vi "init_test_result_table.vi"(10 "Test Table":refnum<vi>, 11 "LED":T1) -> ()   [LabVIEW 2016]
uses:
  <vilib>/Utility/miscctls.llb/LVRowAndColumnTypeDef.ctl
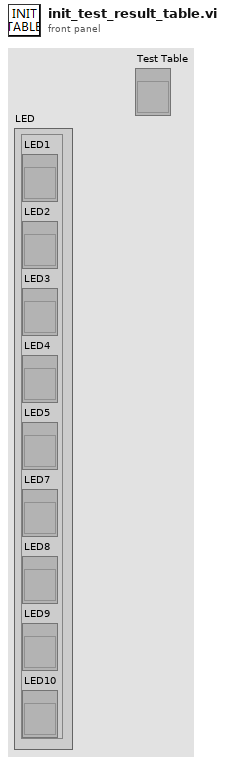
[diagram p1: front panel]
types:
  T1 = cluster{"LED1":refnum<vi>, "LED2":refnum<vi>, "LED3":refnum<vi>, "LED4":refnum<vi>, "LED5":refnum<vi>, "LED7":refnum<vi>, "LED8":refnum<vi>, "LED9":refnum<vi>, "LED10":refnum<vi>}
  T2 = typedef "LVRowAndColumnTypeDef.ctl" = cluster{"Row":i32, "Column":i32}
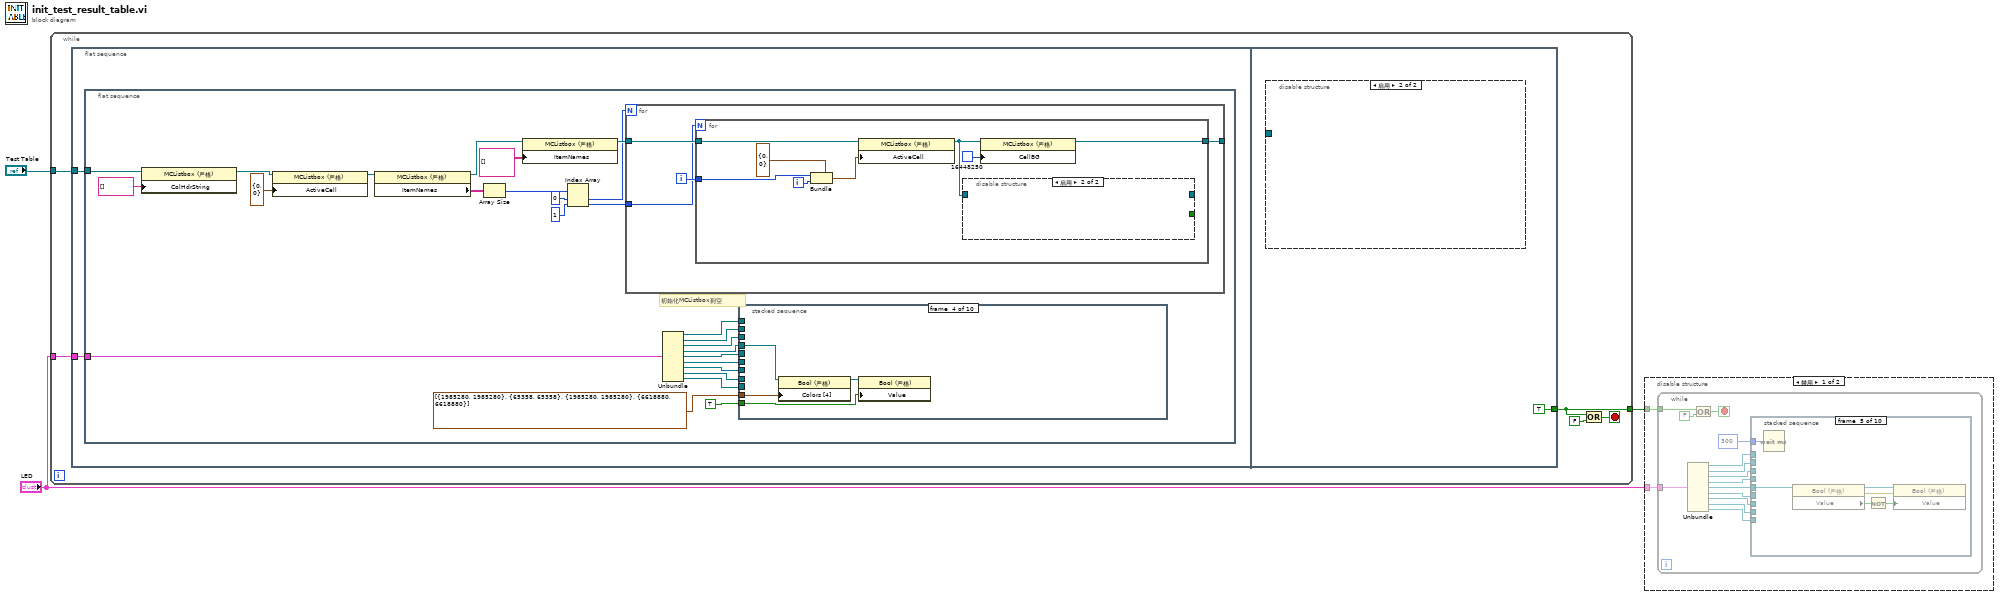
[diagram p0: block diagram]
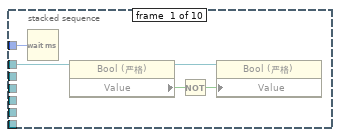
[diagram p2: hidden frame]
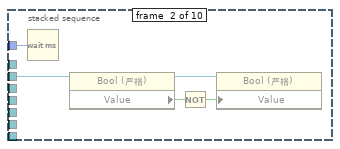
[diagram p3: hidden frame]
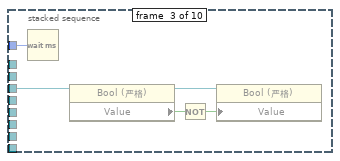
[diagram p4: hidden frame]
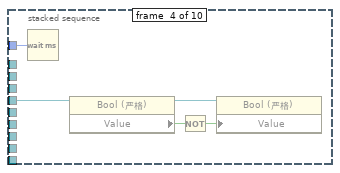
[diagram p5: hidden frame]
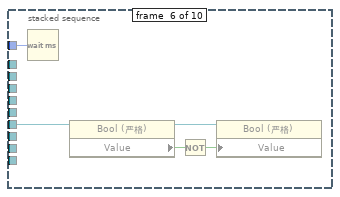
[diagram p6: hidden frame]
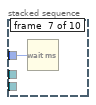
[diagram p7: hidden frame]
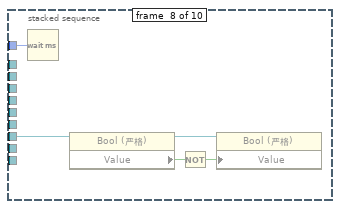
[diagram p8: hidden frame]
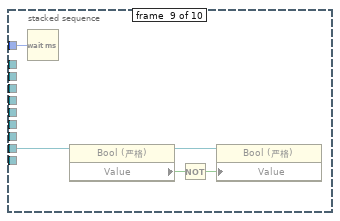
[diagram p9: hidden frame]
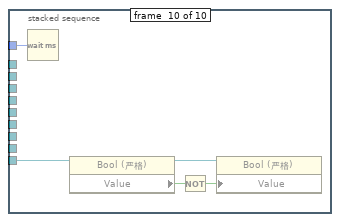
[diagram p10: hidden frame]
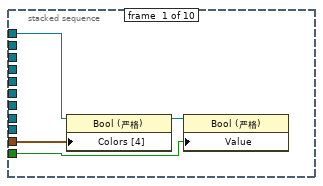
[diagram p12: hidden frame]
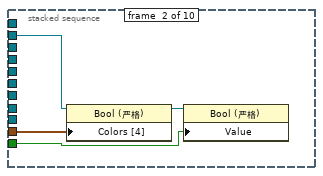
[diagram p13: hidden frame]
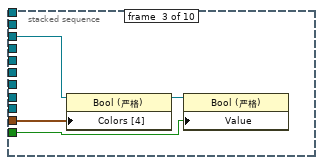
[diagram p14: hidden frame]
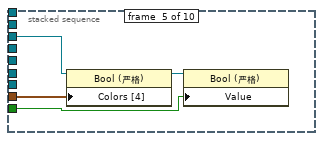
[diagram p15: hidden frame]
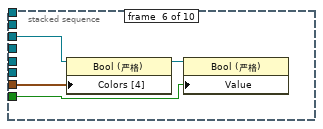
[diagram p16: hidden frame]
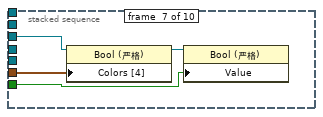
[diagram p17: hidden frame]
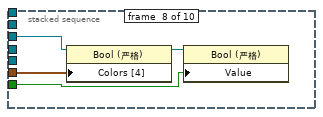
[diagram p18: hidden frame]
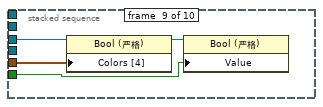
[diagram p19: hidden frame]
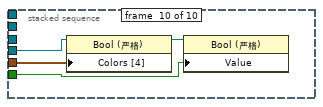
[diagram p20: hidden frame]
diagram:
  n1 = while {
    tunnel: "Test Table" -> [w8]
    tunnel: [w5] -> w3
    tunnel: "LED" -> [w4]
    stop <- w6 stop-if-true
    n2 = flat-sequence {
      tunnel: w8 -> [w9]
      tunnel: w4 -> [w10]
      tunnel: [TRUE] -> w5
      frame #0 {
        n3 = flat-sequence {
          tunnel: w9 -> [w13]
          tunnel: w10 -> [w36]
          frame #0 {
            # "初始化MCListbox到空"
            n4 = property class="MCListbox (严格)"(reference=w13, "ColHdrString"=string[] [] ("列首字符串[]")) -> (reference out=w12:refnum<vi>)  [unwired: 1 in, 1 out]
            n5 = property class="MCListbox (严格)"(reference=w12, "ActiveCell"=T2 {"Row"=0, "Column"=0} ("活动单元格:活动单元格")) -> (reference out=w21:refnum<vi>)  [unwired: 1 in, 1 out]
            n6 = property class="MCListbox (严格)"(reference=w21) -> (reference out=w20:refnum<vi>, "ItemNames"=w19:string[][])  [unwired: 1 in, 1 out]
            n7 = Array Size(array=w19) -> (size(s)=w18:i32[])
            n8 = property class="MCListbox (严格)"(reference=w20, "ItemNames"=string[][] [] ("项名")) -> (reference out=w33:refnum<vi>)  [unwired: 1 in, 1 out]
            n9 = Index Array(array=w18, index #1=0 ("索引"), index #2=1 ("索引")) -> (element #1=w16:i32, element #2=w14:i32)
            n10 = for {
              N: w16 -> [_]
              tunnel: w33 -> [w79]
              tunnel: [w78] -> _
              tunnel: w14 -> [w77]
              i -> [w80]
              n11 = for {
                N: w77 -> [_]
                tunnel: w80 -> [w87]
                tunnel: w79 -> [w84]
                tunnel: [w83] -> w78
                i -> [w86]
                n12 = Bundle(cluster=cluster{i32, i32} {0, 0} ("簇"), w87, w86) -> (w88:cluster{i32, i32})
                n13 = property class="MCListbox (严格)"(reference=w84, "ActiveCell"=w88) -> (reference out=w81:refnum<vi>)  [unwired: 1 in, 1 out]
                n14 = disable-structure shown="启用" {
                  disable-tunnel: w81 -> [w91 _]
                  disable-tunnel: [w90 _] -> _
                  disable-tunnel: [w89 _] -> _
                  frame Disabled {
                    n15 = property class="MCListbox (严格)"(reference=w91) -> (reference out=w90:refnum<vi>, "CellBG"=w92:u32)  [unwired: 1 in, 1 out]
                    n16 = Not Equal?(x=w92) -> (x != y?=w89:bool)  [unwired: 1 in]
                  }
                  frame Enabled {
                  }
                }
                n17 = property class="MCListbox (严格)"(reference=w81, "CellBG"=u32 16448250) -> (reference out=w83:refnum<vi>)  [unwired: 1 in, 1 out]
              }
            }
            n18 = Unbundle(w36) -> ("LED1"=w32:refnum<vi>, "LED2"=w31:refnum<vi>, "LED3"=w30:refnum<vi>, "LED4"=w29:refnum<vi>, "LED5"=w28:refnum<vi>, "LED7"=w27:refnum<vi>, "LED8"=w24:refnum<vi>, "LED9"=w25:refnum<vi>, "LED10"=w26:refnum<vi>)
            n19 = stacked-sequence {
              tunnel: w32 -> [w40 _ _ _ _ _ _ _ _ _]
              tunnel: w31 -> [_ w44 _ _ _ _ _ _ _ _]
              tunnel: w30 -> [_ _ w48 _ _ _ _ _ _ _]
              tunnel: w29 -> [_ _ _ w52 _ _ _ _ _ _]
              tunnel: w28 -> [_ _ _ _ w56 _ _ _ _ _]
              tunnel: w27 -> [_ _ _ _ _ w60 _ _ _ _]
              tunnel: w26 -> [_ _ _ _ _ _ _ _ _ w76]
              tunnel: w25 -> [_ _ _ _ _ _ _ _ w71 _]
              tunnel: w24 -> [_ _ _ _ _ _ w64 w68 _ _]
              tunnel: cluster{u32, u32}[] [{1985280, 1985280}, {65358, 65358}, {1985280, 1985280}, {6618880, 6618880}] ("颜色[4]") -> [w39 w43 w47 w51 w55 w59 w63 w67 w72 w75]
              tunnel: TRUE -> [w38 w42 w46 w49 w53 w57 w61 w65 w69 w73]
              frame #0 {
                n20 = property class="Bool (严格)"(reference=w40, "Colors [4]"=w39) -> (reference out=w37:refnum<vi>)  [unwired: 1 in, 1 out]
                n21 = property class="Bool (严格)"(reference=w37, "Value"=w38) -> ()  [unwired: 1 in, 2 out]
              }
              frame #1 {
                n22 = property class="Bool (严格)"(reference=w44, "Colors [4]"=w43) -> (reference out=w41:refnum<vi>)  [unwired: 1 in, 1 out]
                n23 = property class="Bool (严格)"(reference=w41, "Value"=w42) -> ()  [unwired: 1 in, 2 out]
              }
              frame #2 {
                n24 = property class="Bool (严格)"(reference=w48, "Colors [4]"=w47) -> (reference out=w45:refnum<vi>)  [unwired: 1 in, 1 out]
                n25 = property class="Bool (严格)"(reference=w45, "Value"=w46) -> ()  [unwired: 1 in, 2 out]
              }
              frame #3 {
                n26 = property class="Bool (严格)"(reference=w52, "Colors [4]"=w51) -> (reference out=w50:refnum<vi>)  [unwired: 1 in, 1 out]
                n27 = property class="Bool (严格)"(reference=w50, "Value"=w49) -> ()  [unwired: 1 in, 2 out]
              }
              frame #4 {
                n28 = property class="Bool (严格)"(reference=w56, "Colors [4]"=w55) -> (reference out=w54:refnum<vi>)  [unwired: 1 in, 1 out]
                n29 = property class="Bool (严格)"(reference=w54, "Value"=w53) -> ()  [unwired: 1 in, 2 out]
              }
              frame #5 {
                n30 = property class="Bool (严格)"(reference=w60, "Colors [4]"=w59) -> (reference out=w58:refnum<vi>)  [unwired: 1 in, 1 out]
                n31 = property class="Bool (严格)"(reference=w58, "Value"=w57) -> ()  [unwired: 1 in, 2 out]
              }
              frame #6 {
                n32 = property class="Bool (严格)"(reference=w64, "Colors [4]"=w63) -> (reference out=w62:refnum<vi>)  [unwired: 1 in, 1 out]
                n33 = property class="Bool (严格)"(reference=w62, "Value"=w61) -> ()  [unwired: 1 in, 2 out]
              }
              frame #7 {
                n34 = property class="Bool (严格)"(reference=w68, "Colors [4]"=w67) -> (reference out=w66:refnum<vi>)  [unwired: 1 in, 1 out]
                n35 = property class="Bool (严格)"(reference=w66, "Value"=w65) -> ()  [unwired: 1 in, 2 out]
              }
              frame #8 {
                n36 = property class="Bool (严格)"(reference=w71, "Colors [4]"=w72) -> (reference out=w70:refnum<vi>)  [unwired: 1 in, 1 out]
                n37 = property class="Bool (严格)"(reference=w70, "Value"=w69) -> ()  [unwired: 1 in, 2 out]
              }
              frame #9 {
                n38 = property class="Bool (严格)"(reference=w76, "Colors [4]"=w75) -> (reference out=w74:refnum<vi>)  [unwired: 1 in, 1 out]
                n39 = property class="Bool (严格)"(reference=w74, "Value"=w73) -> ()  [unwired: 1 in, 2 out]
              }
            }
          }
        }
      }
      frame #1 {
        n40 = disable-structure shown="启用" {
          disable-tunnel: _ -> [w94 _]
          frame Disabled {
            n41 = stacked-sequence {
              tunnel: w94 -> [w100 w106]
              tunnel: 100 -> [w97 w103]
              tunnel: [_ w102] -> w95
              frame #0 {
                w99 = TRUE
                n42 = Wait (ms)(milliseconds to wait=w97) -> ()  [unwired: 1 out]
                n43 = Variant To Data(type=w99, Variant=w99) -> (data=w98:bool)  [unwired: 1 in, 1 out]
                n44 = invoke class="VI (严格)" method="Ctrl Val.Set"(reference=w100, "Control Name"="Blinking" ("控件名"), "Value"=w98) -> ()  [unwired: 2 in, 5 out]
              }
              frame #1 {
                w105 = FALSE
                n45 = Wait (ms)(milliseconds to wait=w103) -> ()  [unwired: 1 out]
                n46 = Variant To Data(type=w105, Variant=w105) -> (data=w104:bool)  [unwired: 1 in, 1 out]
                n47 = invoke class="VI (严格)" method="Ctrl Val.Set"(reference=w106, "Control Name"="Blinking" ("控件名"), "Value"=w104) -> (reference out=w102:refnum<vi>)  [unwired: 2 in, 4 out]
              }
            }
            n48 = Close Reference(reference=w95) -> ()  [unwired: 1 in, 1 out]
          }
          frame Enabled {
          }
        }
      }
    }
    n49 = Or(x=w5, y=FALSE) -> (x .or. y?=w6:bool)
  }
  n50 = disable-structure shown="禁用" {
    disable-tunnel: w3 -> [w109 _]
    disable-tunnel: "LED" -> [w108 _]
    frame Disabled {
      n51 = while {
        tunnel: w108 -> [w123]
        tunnel: w109 -> [w112]
        stop <- w111 stop-if-true
        n52 = Unbundle(w123) -> ("LED1"=w122:refnum<vi>, "LED2"=w120:refnum<vi>, "LED3"=w119:refnum<vi>, "LED4"=w118:refnum<vi>, "LED5"=w117:refnum<vi>, "LED7"=w116:refnum<vi>, "LED8"=w113:refnum<vi>, "LED9"=w114:refnum<vi>, "LED10"=w115:refnum<vi>)
        n53 = Or(x=w112, y=FALSE) -> (x .or. y?=w111:bool)
        n54 = stacked-sequence {
          tunnel: w122 -> [w128 _ _ _ _ _ _ _ _ _]
          tunnel: 300 -> [w124 w131 w134 w139 w145 w152 w155 w158 w161 w168]
          tunnel: w120 -> [_ w133 _ _ _ _ _ _ _ _]
          tunnel: w119 -> [_ _ w135 _ _ _ _ _ _ _]
          tunnel: w118 -> [_ _ _ w143 _ _ _ _ _ _]
          tunnel: w117 -> [_ _ _ _ w144 _ _ _ _ _]
          tunnel: w116 -> [_ _ _ _ _ w151 _ _ _ _]
          tunnel: w115 -> [_ _ _ _ _ _ _ _ _ w170]
          tunnel: w114 -> [_ _ _ _ _ _ _ _ w165 _]
          tunnel: w113 -> [_ _ _ _ _ _ _ w160 _ _]
          frame #0 {
            n55 = Wait (ms)(milliseconds to wait=w124) -> ()  [unwired: 1 out]
            n56 = property class="Bool (严格)"(reference=w128) -> (reference out=w127:refnum<vi>, "Value"=w126:bool)  [unwired: 1 in, 1 out]
            n57 = Not(x=w126) -> (.not. x?=w125:bool)
            n58 = property class="Bool (严格)"(reference=w127, "Value"=w125) -> ()  [unwired: 1 in, 2 out]
          }
          frame #1 {
            n59 = Wait (ms)(milliseconds to wait=w131) -> ()  [unwired: 1 out]
            n60 = property class="Bool (严格)"(reference=w133) -> (reference out=w132:refnum<vi>, "Value"=w130:bool)  [unwired: 1 in, 1 out]
            n61 = Not(x=w130) -> (.not. x?=w129:bool)
            n62 = property class="Bool (严格)"(reference=w132, "Value"=w129) -> ()  [unwired: 1 in, 2 out]
          }
          frame #2 {
            n63 = Wait (ms)(milliseconds to wait=w134) -> ()  [unwired: 1 out]
            n64 = property class="Bool (严格)"(reference=w135) -> (reference out=w136:refnum<vi>, "Value"=w138:bool)  [unwired: 1 in, 1 out]
            n65 = Not(x=w138) -> (.not. x?=w137:bool)
            n66 = property class="Bool (严格)"(reference=w136, "Value"=w137) -> ()  [unwired: 1 in, 2 out]
          }
          frame #3 {
            n67 = Wait (ms)(milliseconds to wait=w139) -> ()  [unwired: 1 out]
            n68 = property class="Bool (严格)"(reference=w143) -> (reference out=w142:refnum<vi>, "Value"=w141:bool)  [unwired: 1 in, 1 out]
            n69 = Not(x=w141) -> (.not. x?=w140:bool)
            n70 = property class="Bool (严格)"(reference=w142, "Value"=w140) -> ()  [unwired: 1 in, 2 out]
          }
          frame #4 {
            n71 = Wait (ms)(milliseconds to wait=w145) -> ()  [unwired: 1 out]
            n72 = property class="Bool (严格)"(reference=w144) -> (reference out=w149:refnum<vi>, error out=w148:errorcluster, "Value"=w147:bool)  [unwired: 1 in]
            n73 = Not(x=w147) -> (.not. x?=w146:bool)
            n74 = property class="Bool (严格)"(reference=w149, error in=w148, "Value"=w146) -> ()  [unwired: 2 out]
          }
          frame #5 {
            n75 = Wait (ms)(milliseconds to wait=w152) -> ()  [unwired: 1 out]
            n76 = property class="Bool (严格)"(reference=w151) -> (reference out=w150:refnum<vi>, "Value"=w154:bool)  [unwired: 1 in, 1 out]
            n77 = Not(x=w154) -> (.not. x?=w153:bool)
            n78 = property class="Bool (严格)"(reference=w150, "Value"=w153) -> ()  [unwired: 1 in, 2 out]
          }
          frame #6 {
            n79 = Wait (ms)(milliseconds to wait=w155) -> ()  [unwired: 1 out]
          }
          frame #7 {
            n80 = Wait (ms)(milliseconds to wait=w158) -> ()  [unwired: 1 out]
            n81 = property class="Bool (严格)"(reference=w160) -> (reference out=w159:refnum<vi>, "Value"=w157:bool)  [unwired: 1 in, 1 out]
            n82 = Not(x=w157) -> (.not. x?=w156:bool)
            n83 = property class="Bool (严格)"(reference=w159, "Value"=w156) -> ()  [unwired: 1 in, 2 out]
          }
          frame #8 {
            n84 = Wait (ms)(milliseconds to wait=w161) -> ()  [unwired: 1 out]
            n85 = property class="Bool (严格)"(reference=w165) -> (reference out=w164:refnum<vi>, "Value"=w163:bool)  [unwired: 1 in, 1 out]
            n86 = Not(x=w163) -> (.not. x?=w162:bool)
            n87 = property class="Bool (严格)"(reference=w164, "Value"=w162) -> ()  [unwired: 1 in, 2 out]
          }
          frame #9 {
            n88 = Wait (ms)(milliseconds to wait=w168) -> ()  [unwired: 1 out]
            n89 = property class="Bool (严格)"(reference=w170) -> (reference out=w169:refnum<vi>, "Value"=w167:bool)  [unwired: 1 in, 1 out]
            n90 = Not(x=w167) -> (.not. x?=w166:bool)
            n91 = property class="Bool (严格)"(reference=w169, "Value"=w166) -> ()  [unwired: 1 in, 2 out]
          }
        }
      }
    }
    frame Enabled {
    }
  }
